vi "ControlFunction.vi"(8 "error in (no error)":errorcluster, 11 "Drive in":refnum<class "Drive.lvclass">) -> (0 "error out":errorcluster, 3 "Drive out":refnum<class "Drive.lvclass">)   [LabVIEW 2017, in "Drive.lvclass"]
uses:
  Drive.lvclass
  <vilib>/Rock Robotics/WPI/ThirdParty/Phoenix-LabVIEW/Motor Controller/Controls/CTRE_Phoenix_MotorControl_ControlMode.ctl
  SubsystemData/DriveData/DriveOutput.ctl
  SubsystemData/DriveData/DriveData.lvclass
  R:/Documents/github/FRC4080/2018-robot-main/SubsystemData/SubsystemData.lvclass
  Drive.lvclass/Drive.ctl
  <vilib>/Rock Robotics/WPI/Joystick/WPI_JoystickTankMapping.vi
  SubsystemData/SubsystemData.lvclass
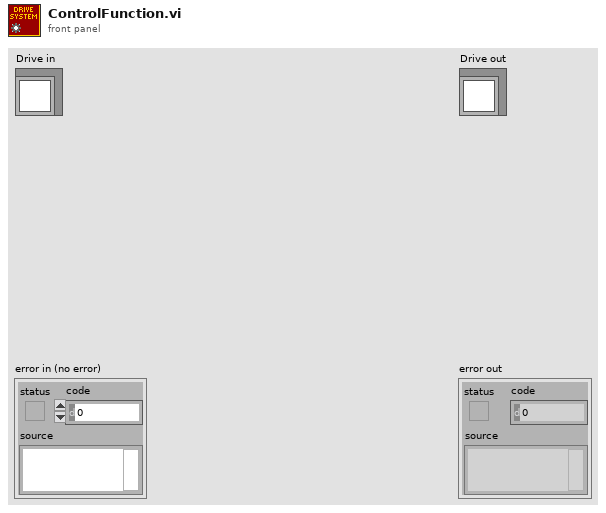
[diagram p1: front panel]
types:
  T1 = typedef "DriveData.lvclass/DriveOutput.ctl" = cluster{"LeftDriveSetting":dbl, "RightDriveSetting":dbl, "Control Mode":T2}
  T2 = typedef "CTRE_Phoenix_MotorControl_ControlMode.ctl" = u16
  T3 = typedef "DriveData.lvclass/DriveCommand.ctl" = cluster{"RightDriveMagnatude":dbl, "LeftDriveMagnatude":dbl}
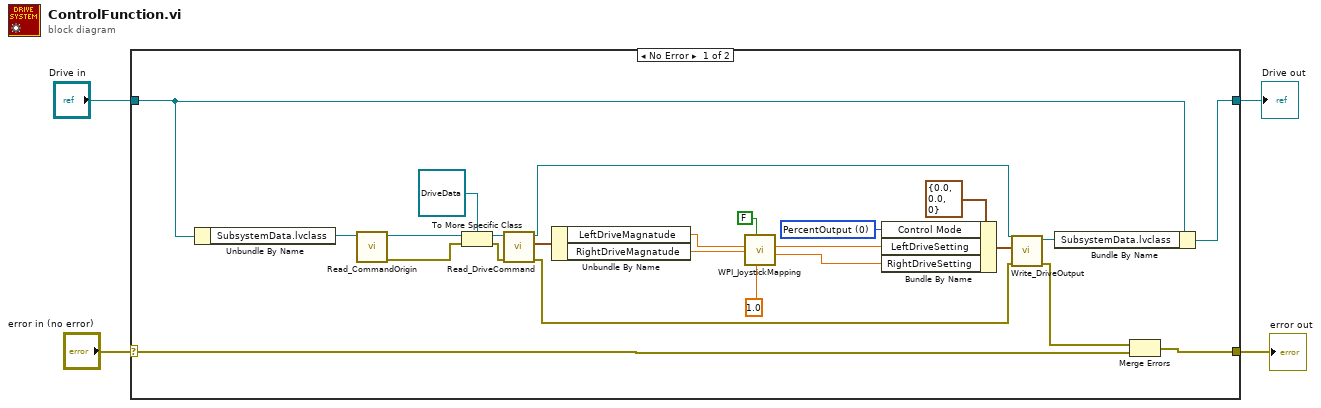
[diagram p0: block diagram]
diagram:
  n1 = case shown="No Error" "error in (no error)" {
    selector: "error in (no error)" -> [w8 w29]
    tunnel: "Drive in" -> [w13 w30]
    tunnel: [w12 w30] -> w3
    tunnel: [w6 w29] -> w1
    frame No Error {
      w22 = T2 0 items=["PercentOutput"=0, "Position"=1, "Velocity"=2, "Current"=3, "Follower"=5, "MotionProfile"=6, "MotionMagic"=7, "MotionMagicArc"=8, "MotionProfileArc"=10, "Disabled"=15] ("Control Mode")
      n2 = Unbundle By Name(w13) -> ("SubsystemData.lvclass"=w21:refnum<class "SubsystemData.lvclass">)
      n3 = call-dynamic "Read_CommandOrigin.vi"("SubsystemData in"=w21) -> ("error out"=w16:errorcluster, "SubsystemData out"=w19:refnum<class "SubsystemData.lvclass">)  [unwired: 8 in, 1 out]
      n4 = To More Specific Class(target class=refnum<class "DriveData.lvclass"> refnum ("DriveData out"), reference=w19, error in=w16) -> (specific class reference=w18:refnum<class "DriveData.lvclass">, error out=w20:errorcluster)
      n5 = call-dynamic "Read_DriveCommand.vi"("error in (no error)"=w20, "DriveData in"=w18) -> ("error out"=w7:errorcluster, "DriveCommand"=w11:T3, "DriveData out"=w15:refnum<class "DriveData.lvclass">)  [unwired: 7 in]
      n6 = Unbundle By Name(w11) -> ("LeftDriveMagnatude"=w9:dbl, "RightDriveMagnatude"=w10:dbl)
      n7 = call-poly <vilib>:"WPI_JoystickMapping.vi"("Max Output"=1.0, "Square Inputs"=FALSE, "Right axis value"=w10, "Left axis value"=w9) -> ("Right Motor Value"=w23:dbl, "Left Motor Value"=w24:dbl)  [unwired: 6 in]
      n8 = Bundle By Name(cluster=T1 {"LeftDriveSetting"=0.0, "RightDriveSetting"=0.0, "Control Mode"=0} ("DriveOutput"), "Control Mode"=w22, "LeftDriveSetting"=w24, "RightDriveSetting"=w23) -> (w26:T1)
      n9 = call-dynamic "Write_DriveOutput.vi"("error in (no error)"=w7, "DriveOutput"=w26, "DriveData in"=w15) -> ("error out"=w5:errorcluster, "DriveData out"=w14:refnum<class "DriveData.lvclass">)  [unwired: 7 in]
      n10 = Bundle By Name(cluster=w13, "SubsystemData.lvclass"=w14) -> (w12:refnum<class "Drive.lvclass">)
      n11 = Merge Errors(w5, w8) -> (w6:errorcluster)
    }
    frame Error {
    }
  }
  "error out" <- w1
  "Drive out" <- w3
